vi "Main_Stagefright LIVE.vi"() -> ()   [LabVIEW 2012]
uses:
  <vilib>/userdefined/High Color/IMAQdx.ctl
  <vilib>/vision/Image Controls.llb/IMAQ Image.ctl
  <vilib>/vision/NI_Vision_Development_Module.lvlib
  <vilib>/vision/driver/NI_Vision_Acquisition_Software.lvlib
panel:
  in  "reset count":bool
  out "Count":u32=29
  out "Score":sgl format="%#.0f"
  out "Y (pixel)":sgl format="%.1f"
  out "X (pixel)":sgl format="%.1f"
  out "Angle (deg)":sgl format="%.1f"
  out "Version":string
  in  "Filename":string
  in  "Export Folder":path
  in  "Save results to CSV":bool
  out "Processing Time (ms)":u32=29
  in  "Camera":T1="cam1"
  in  "start":bool
  out "Fiducial Template":T2(plugin-control)
  in  "Fiducial File Path":path=path "C:/Users/kevinsh/Desktop/Stage Fright SVN/Data/Template_StageFrightChip_20x.png"
  in  "stop":bool
  in  "Minimum Match Score":sgl=600.0
  in  "Search Angle Range":cluster{"Start (deg)":sgl, "End (deg)":sgl}[](array[cluster])=[{"Start (deg)"=-15.0, "End (deg)"=15.0}]
  out "Live Image":T2(plugin-control)
  # "Match Results"
  # "LIVE"
  # "Data Export"
  # "Setup"
  # "Search Settings"
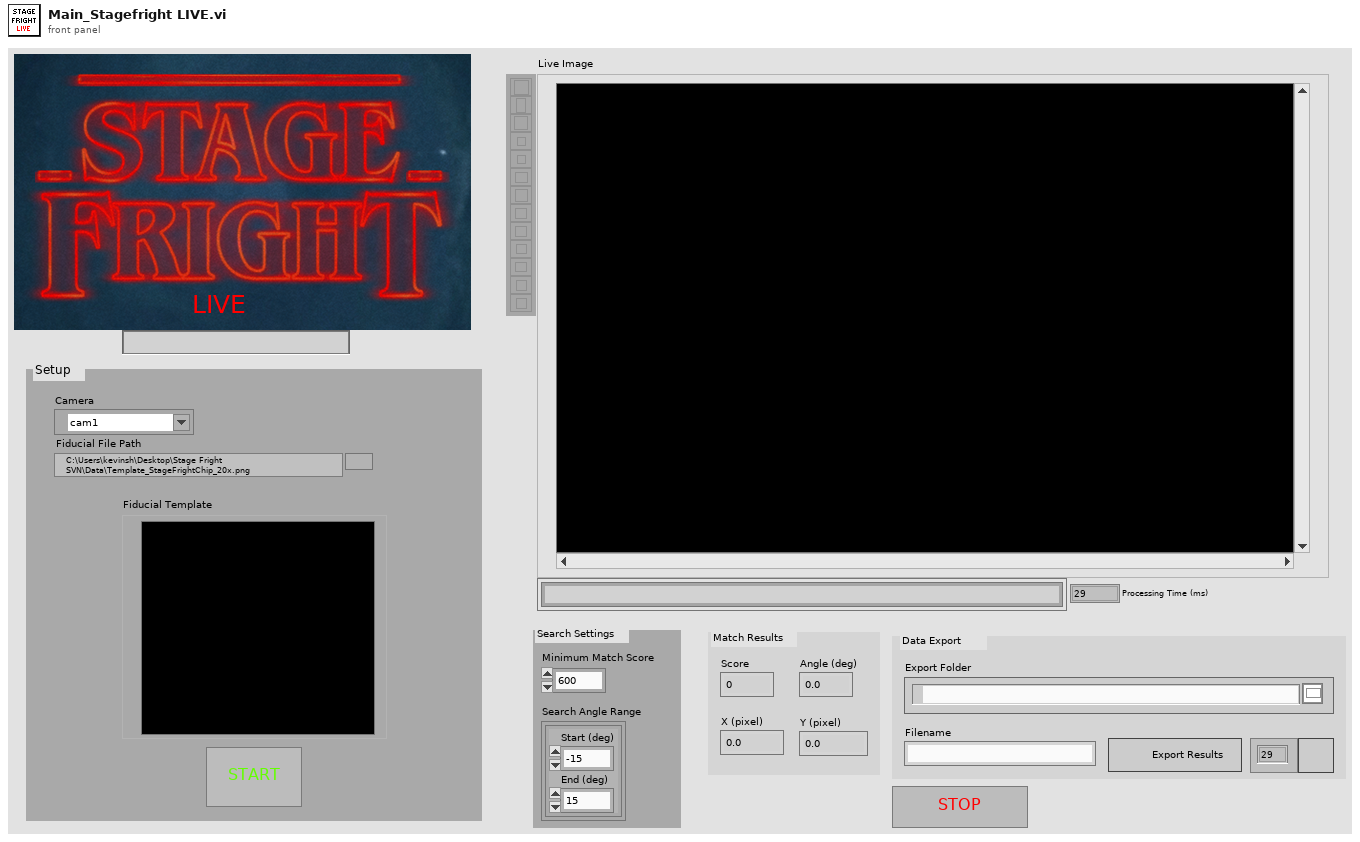
[diagram p1: front panel]
types:
  T1 = typedef "IMAQdx.ctl" = refnum<k21>
  T2 = typedef "IMAQ Image.ctl" = refnum<image>
  T3 = typedef "Image Type" = u32
  T4 = cluster{"Match Mode":u16, "Number of Matches Requested":i32, "Minimum Match Score":sgl, "SubPixel Accuracy":bool, "Rotation Angle Ranges":cluster{"Start":sgl, "End":sgl}[], "Show Search Area":bool, "Show Result":bool}
  T5 = cluster{"Position":cluster{"x":sgl, "y":sgl}, "Angle":sgl, "Scale":sgl, "Score":sgl, "Bounding Box":cluster{"x":sgl, "y":sgl}[]}[]
  T6 = cluster{"Position":cluster{"x":sgl, "y":sgl}, "Angle":sgl, "Scale":sgl, "Score":sgl, "Bounding Box":cluster{"x":sgl, "y":sgl}[]}
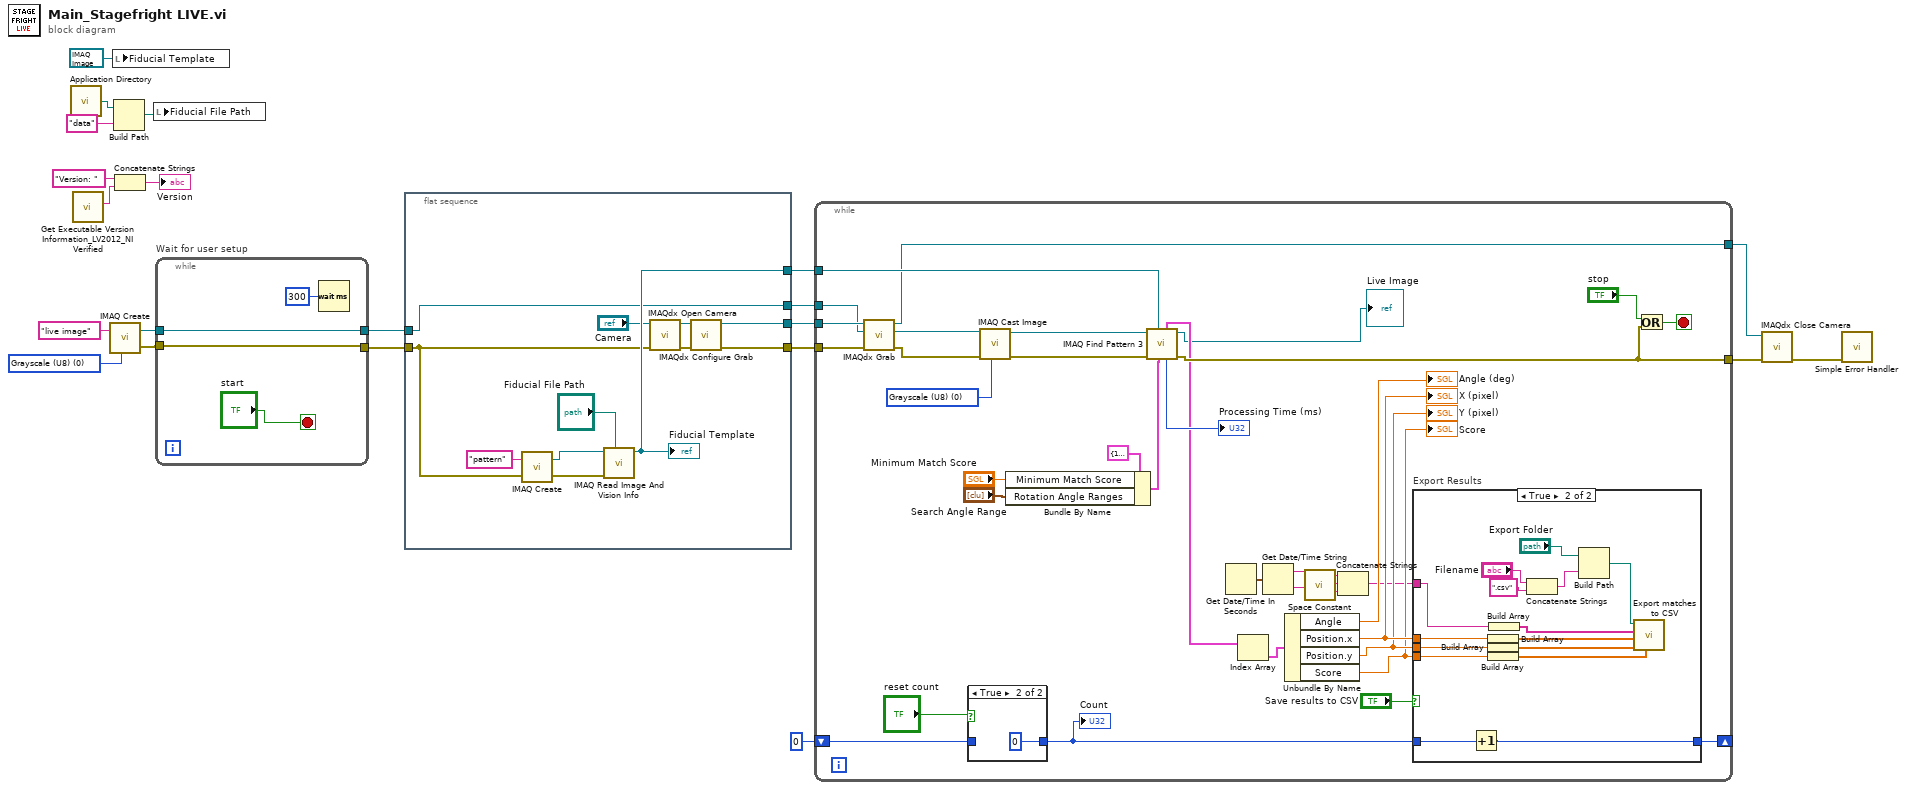
[diagram p0: block diagram]
diagram:
  w11 = T3 0 items=["Grayscale (U8)", "Grayscale (I16)", "Grayscale (SGL)", "Complex (CSG)", "RGB (U32)", "HSL (U32)", "RGB (U64)", "Grayscale (U16)"] ("Image Type")
  n1 = call <vilib>:"Application Directory.vi"() -> ("Application Directory"=w2:path)
  n2 = call "Get Executable Version Information_LV2012_NI Verified.vi"() -> ("FileVersion"=w15:string)  [unwired: 10 in, 1 out]
  n3 = call "IMAQ Create"("Image Name"="live image", "Image Type"=w11) -> ("New Image"=w6:T2, "error out"=w7:errorcluster)  [unwired: 3 in]
  n4 = local write "Fiducial Template"(T2 refnum ("Fiducial Template")) -> ()
  n5 = Build Path(base path=w2, name or relative path="data") -> (appended path=w3:path)
  n6 = Concatenate Strings("Version: " ("string"), w15) -> (→"Version":string)
  n7 = local write "Fiducial File Path"(w3) -> ()
  n8 = while "Wait for user setup" {
    tunnel: [w23] -> w21
    tunnel: w7 -> [w23]
    tunnel: [w22] -> w12
    tunnel: w6 -> [w22]
    stop <- "start" stop-if-true
    n9 = Wait (ms)(milliseconds to wait=u32 300) -> ()  [unwired: 1 out]
  }
  n10 = flat-sequence {
    tunnel: w21 -> [w27]
    tunnel: [w33] -> w20
    tunnel: [w26] -> w19
    tunnel: [w29] -> w18
    tunnel: [w28] -> w17
    tunnel: w12 -> [w26]
    frame #0 {
      n11 = call "IMAQ Create"("Image Name"="pattern", "error in (no error)"=w27) -> ("New Image"=w36:T2, "error out"=w34:errorcluster)  [unwired: 3 in]
      n12 = call "IMAQ Read Image And Vision Info"("File Path"="Fiducial File Path", "error in (no error)"=w34, "Image"=w36) -> ("Image Out"=w33:T2)  [unwired: 1 in, 7 out]
      "Fiducial Template" <- w33
      n13 = call <vilib>:"IMAQdx Open Camera.vi"("error in"=w27, "Session In"="Camera") -> ("error out"=w31:errorcluster, "Session Out"=w30:T1)  [unwired: 1 in, 7 out]
      n14 = call <vilib>:"IMAQdx Configure Grab.vi"("error in"=w31, "Session In"=w30) -> ("error out"=w29:errorcluster, "Session Out"=w28:T1)  [unwired: 8 out]
    }
  }
  n15 = while {
    tunnel: [w60] -> w10
    tunnel: w20 -> [w58]
    tunnel: w19 -> [w62]
    tunnel: w18 -> [w64]
    tunnel: w17 -> [w63]
    tunnel: [w42] -> w8
    shift-right: [w41] -> _
    shift-left: u32 0 ("Count") -> [w40]
    stop <- w59 stop-if-true
    w51 = T3 0 items=["Grayscale (U8)", "Grayscale (I16)", "Grayscale (SGL)", "Complex (CSG)", "RGB (U32)", "HSL (U32)", "RGB (U64)", "Grayscale (U16)"] ("Image Type")
    n16 = call <vilib>:"IMAQdx Grab.vi"("error in"=w64, "Image In"=w62, "Session In"=w63) -> ("error out"=w53:errorcluster, "Image Out"=w55:T2, "Session Out"=w42:T1)  [unwired: 5 in, 1 out]
    n17 = case shown="True" "reset count" {
      tunnel: [w73 u32 0 ("Count")] -> w39
      tunnel: w40 -> [w73 _]
      frame False {
      }
      frame True {
      }
    }
    "Count" <- w39
    n18 = call "IMAQ Cast Image"("Image Type"=w51, "error in (no error)"=w53, "Image Src"=w55) -> ("error out"=w52:errorcluster, "Image Dst Out"=w54:T2)  [unwired: 7 in]
    n19 = Bundle By Name(cluster=T4 {"Match Mode"=1, "Number of Matches Requested"=1, "Minimum Match Score"=800.0, "SubPixel Accuracy"=TRUE, "Rotation Angle Ranges"=[], "Show Search Area"=FALSE, "Show Result"=TRUE} ("Settings"), "Minimum Match Score"="Minimum Match Score", "Rotation Angle Ranges"="Search Angle Range") -> (w65:T4)
    n20 = call "IMAQ Find Pattern 3"("Settings"=w65, "Template"=w58, "error in (no error)"=w52, "Image"=w54) -> ("error out"=w60:errorcluster, "Image Out"=→"Live Image":T2, "Elapsed time (ms)"=→"Processing Time (ms)":u32, "Matches"=w56:T5)  [unwired: 2 in, 2 out]
    n21 = Get Date/Time In Seconds() -> (seconds since 1Jan1904=w46:timestamp)
    n22 = Index Array(array=w56) -> (element=w48:T6)  [unwired: 1 in]
    n23 = Get Date/Time String(seconds (now)=w46) -> (date string=w47:string, time string=w44:string)  [unwired: 2 in]
    n24 = Unbundle By Name(w48) -> ("Angle"=→"Angle (deg)":sgl, "Position.x"=w72:sgl, "Position.y"=w71:sgl, "Score"=w70:sgl)
    "X (pixel)" <- w72
    "Y (pixel)" <- w71
    "Score" <- w70
    n25 = call <vilib>:"Space Constant.vi"() -> ("String"=w43:string)
    n26 = Concatenate Strings(w47, w43, w44) -> (w45:string)
    n27 = case "Export Results" shown="True" "Save results to CSV" {
      tunnel: w70 -> [_ w88]
      tunnel: w72 -> [_ w90]
      tunnel: w71 -> [_ w89]
      tunnel: w45 -> [_ w84]
      tunnel: [w75 w76] -> w41
      tunnel: w39 -> [w75 w77]
      frame False {
      }
      frame True {
        n28 = Increment(x=w77) -> (x+1=w76:u32)
        n29 = Build Array(w90) -> (w87:sgl[])
        n30 = Build Array(w89) -> (w85:sgl[])
        n31 = Build Array(w88) -> (w86:sgl[])
        n32 = Build Array(w84) -> (w83:string[])
        n33 = Concatenate Strings("Filename", ".csv" ("string")) -> (w80:string)
        n34 = Build Path(base path="Export Folder", name or relative path=w80) -> (appended path=w78:path)
        n35 = call "Export matches to CSV.vi"("Score"=w86, "PosY"=w85, "PosX"=w87, "filenames for processing"=w83, "Data Export Filepath"=w78) -> ()  [unwired: 7 in]
      }
    }
    n36 = Or(x="stop", y=w60) -> (x .or. y?=w59:bool)
  }
  n37 = call <vilib>:"IMAQdx Close Camera.vi"("error in"=w10, "Session In"=w8) -> ("error out"=w9:errorcluster)  [unwired: 9 in]
  n38 = call <vilib>:"Simple Error Handler.vi"("error in (no error)"=w9) -> ()  [unwired: 4 in, 5 out]
